vi "IMP (SubVI).vi"(6 "Initial Conditions in":dbl[](array[numeric]), 7 "b":dbl[](array[numeric]), 9 "n in":i32[](array[numeric]), 10 "Numeric":i32, 11 "Шаг h, с":dbl) -> (3 "Initial Conditions out":dbl[][](array[numeric]))   [LabVIEW 2016]
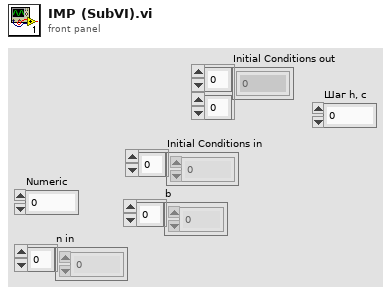
[diagram p1: front panel]
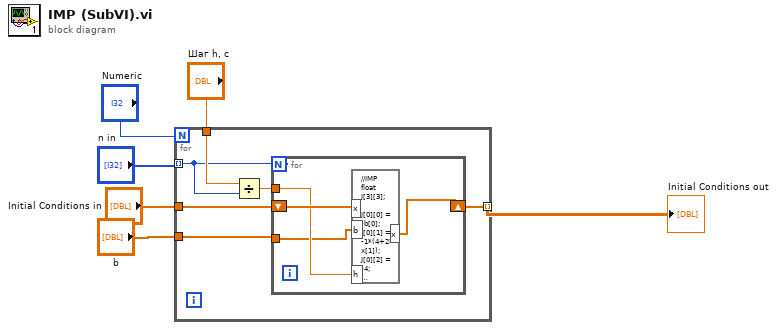
[diagram p0: block diagram]
diagram:
  n1 = for {
    N: "Numeric" -> [_]
    tunnel: "n in" -> [w9] mode=indexing
    tunnel: "Шаг h, с" -> [w12]
    tunnel: "Initial Conditions in" -> [w11]
    tunnel: [w8] -> w1 mode=indexing
    tunnel: "b" -> [w7]
    n2 = Divide(x=w12, y=w9) -> (x/y=w10:dbl)
    n3 = for {
      N: w9 -> [_]
      tunnel: w10 -> [w15]
      shift-right: [w14] -> w8
      shift-left: w11 -> [w16]
      tunnel: w7 -> [w13]
      n4 = formula code="//IMP\nfloat J[3][3];\n\nJ[0][0] = -b[0]; \nJ[0][1] = -1*(4+2*x[1]); \nJ[0][2] = -4; \n\nJ[1][0] = -4; \nJ[1][1] = -b[1];\nJ[1][2] = -1*(4+2*x[2]);\n\nJ[2][0] = -1*(4+2*x[0]); \nJ[2][1] = -4;\nJ[2][2] = -b[2];\n\n\nfloat w[3][4], Z[3], a[3], Zn[3], dz;\nfloat tol;\nint k; int i; int j; float t; float d;\ntol = 1e-14;\nint nnewtmax = 3, nnewt;\ndz = 2e-13;\nnnewt = 0;\n\nZ[0] = x[0]; Z[1] = x[1]; Z[2] = x[2];\nwhile ( (dz > tol) && (nnewt < nnewtmax)){\n\tfor(i=0;i<3;i++)\n\t{\n\t\tfor(j=0;j<3;j++)\n\t\t{\n\t\t\tif (i==j)\n\t\t\tw[i][j]=1 - 0.5*h*J[i][j];\n\t\t\telse\n\t\t\tw[i][j]= - 0.5*h*J[i][j];\n\t\t}\n\t}\n\n\n\n\ta[0] = 0.5*(x[0] + Z[0]);\n\ta[1] = 0.5*(x[1] + Z[1]);\n\ta[2] = 0.5*(x[2] + Z[2]);\n\t\n\tw[0][3]= -Z[0]+x[0]+h*(-b[0]*a[0]-4*(a[1]+a[2])-a[1]*a[1]);\n\tw[1][3]= -Z[1]+x[1]+h*(-b[1]*a[1]-4*(a[0]+a[2])-a[2]*a[2]);\n\tw[2][3]= -Z[2]+x[2]+h*(-b[2]*a[2]-4*(a[1]+a[0])-a[0]*a[0]);\n\t\n\t\n\tfor(k = 0; k <= 1; k++){\n\t\tint l = k;\n\t\n\t\tfor( i = k+1; i<= 2; i++){\n\t\t\tif( abs(w[i][k]) > abs(w[l][k]) ){\n\t\t\tl = i;\n\t\t\t}\n\t\t}\n\t\tif (l != k){\n\t\t\tfor( j = 0; j <= 3; j++){\n\t\t\t\tif ((j == 0) || (j >= k)){\n\t\t\t\t\tt = w[k][j];\n\t\t\t\t\tw[k][j] = w[l][j];\n\t\t\t\t\tw[l][j] = t;\n\t\t\t\t}\n\t\t\t}\n\t\t}\t\n\n\t\td = 1.0 / w[k][k];\n\t\tfor( i=(k+1); i <=(2); i++){\n\t\t\tif (w[i][k] == 0){\n\t\t\t\tcontinue;\n\t\t\t}\n\t\t\tt = w[i][k] * d;\n\t\t\tfor ( j = k; j <= (3); j++) {\n\t\t\t\tif (w[k][j] != 0){\n\t\t\t\t\tw[i][j] = w[i][j] - t * w[k][j];\n\t\t\t\t}\n\t\t\t}\n\t\t}\n\t}\n\tfor( i=(3); i >= 2; i--){\n\t\tfor( j=1; j <= i-1; j++){\n\t\t\tt = w[i - j - 1][i - 1]/w[ i -1][i - 1];\n\t\t\tw[i-j - 1][ 3] = w[i-j -1][3] - t*w[i - 1][ 3];\n\t\t}\n\t\tw[i-1][ 3] = w[i - 1][3]/w[ i -1][i - 1];\n\t}\n\tw[0][3] = w[0][3]/w[0][0];\n\tZn[0] = Z[0]+ w[0][3];\n\tZn[1] = Z[1]+ w[1][3];\n\tZn[2] = Z[2]+ w[2][3];\n\t\n\tdz = ( (Zn[0] - Z[0])**2 + (Zn[1] - Z[1])**2 + (Zn[2] - Z[2])**2 )**0.5;\n\tZ[0] = Zn[0];\n\tZ[1] = Zn[1];\n\tZ[2] = Zn[2];\n\n\tnnewt ++;\n}\n\nx[0] = Zn[0];\nx[1] = Zn[1];\nx[2] = Zn[2];"("x"=w16, "h"=w15, "b"=w13) -> ("x"=w14:dbl[])
    }
  }
  "Initial Conditions out" <- w1
